vi "Red Pitaya Manager.vi"() -> ()   [LabVIEW 2024]
uses:
  Libraries/Red Pitaya/RP Core/RP Communicator/RP Communicator.lvclass
  <vilib>/regexp/Match Regular Expression.xnode
  Libraries/Red Pitaya/Red Pitaya Digitizer/Red Pitaya Digitizer.lvclass
  Libraries/Red Pitaya/RP Command.ctl
  Libraries/Red Pitaya/RP Status Offsets.ctl
  Libraries/Red Pitaya/RP Config Offsets.ctl
  Libraries/Red Pitaya/RP Channel Calibration.ctl
  Libraries/Red Pitaya/RP Calibration 4ch.ctl
  Libraries/Red Pitaya/RP Channel Filter.ctl
  Libraries/Red Pitaya/RP Filter 4ch.ctl
  Libraries/Red Pitaya/RP Calibration 2ch.ctl
  Libraries/Red Pitaya/RP Calibration.ctl
panel:
  in  "minimized shell":bool
  in  "Find Red Pitayas":bool
  out "Calibration":T1
  out "output cluster":T1
  in  "Tab Control":enum32{"Manage", "Settings", "Diagnostics"}(tab)
  out "String":string
  in  "Calibration string":bool
  in  "Applied \nvoltage":dbl=0.5
  in  "Auto gains":bool
  in  "Auto offsets":bool
  in  "Out amplitude":dbl[](array[numeric])=[0.5, 0.5]
  in  "Frequencies":dbl[](array[numeric])=[0.0, 0.0] format="%#_6pHz"
  in  "Out enable":bool[](array[boolean])
  in  "Out gains":dbl[](array[numeric])=[1.0, 1.0]
  in  "Out offsets":i16[](array[numeric])=[0, 0]
  in  "Reset calibration":bool
  out "Waveform Chart":dbl[][](graph)
  in  "Input ranges":bool[](array[boolean])=[FALSE, FALSE, FALSE, FALSE]
  in  "In offsets":i32[](array[numeric])
  in  "In gains":dbl[](array[numeric])
  out "Calibrating":bool
  in  "Write callibration":bool
  in  "Stop calibration":bool
  in  "Start calibration":bool
  out "Starup script":string
  in  "View  startup":bool
  in  "View  bitfiles":bool
  in  "Red Pitayas":i32(listbox)
  out "bit files":string
  in  "bitfile functionality":string[](array[string])=["variable-rate digitizer", "lockin-digitizer", "slow lockin-digitizer", "lockin-digitizer  for 122.88", "fast 4-ch digitizer", "critical current", "slow critical current", "variable rate 4-ch digitizer", "slow I-V v.7020"]
  in  "Bitfile logic tags 2":u16[](array[numeric])=[152, 159, 164, 169, 157, 154, 155, 158, 156]
  in  "Subnet":string="192.168.1"
  in  "Start address":i32=100
  in  "End address":i32=123
  in  "Bitfile logic tags":u16[](array[numeric])=[101, 102, 109, 113, 152, 154, 155, 156, 157, 158, 159, 164, 169]
  in  "Timeout":i32=100
  out "Bitfile IDs map":map{u16, string}(c390)={152="variable-rate digitizer", 154="critical current", 155="slow critical current", 157="fast 4-ch digitizer", 159="lockin-digitizer", 164="slow lockin-digitizer", 169="lockin-digitizer  for 122.88"}
  out "Addresses":string[](array[string])
  out "Device names":string[](array[string])
  out "Modules":i32[](array[numeric])
  out "DDS modula out":i64[](array[numeric])=[101, 102]
  out "Logic tags out":u16[](array[numeric])=[101, 102]
  out "command":string
  in  "error in":errorcluster
  out "error out":errorcluster
  in  "Exit Button":bool
  # "Input calibration"
  # "Output calibration"
  # "typedef enum {\n    STEM_125_10_v1_0            = 0,\n    STEM_125_14_v1_0            = 1,\n    STEM_125_14_v1_1            = 2,\n    STEM_122_16SDR_v1_0         = 3,\n    STEM_122_16SDR_v1_1         = 4,\n    STEM_125_14_LN_v1_1         = 5,\n    STEM_125_14_Z7020_v1_0      = 6,\n    STEM_125_14_Z7020_LN_v1_1   = 7,\n    STEM_125_14_Z7020_4IN_v1_0  = 8,\n    STEM_125_14_Z7020_4IN_v1_2  = 9,\n    STEM_125_14_Z7020_4IN_v1_3  = 10,\n    STEM_250_12_v1_0            = 11,\n    STEM_250_12_v1_1            = 12,\n    STEM_250_12_v1_2            = 13,\n    STEM_250_12_120             = 14,\n    STEM_250_12_v1_2a           = 15,\n    STEM_250_12_v1_2b           = 16,\n    STEM_125_14_LN_BO_v1_1      = 17,\n    STEM_125_14_LN_CE1_v1_1     = 18,\n    STEM_125_14_LN_CE2_v1_1     = 19\n}  rp_HPeModels_t;"
  # "typedef enum {\n    Z7010 = 0,\n    Z7020 = 1\n}  rp_HPeZynqModels_t;"
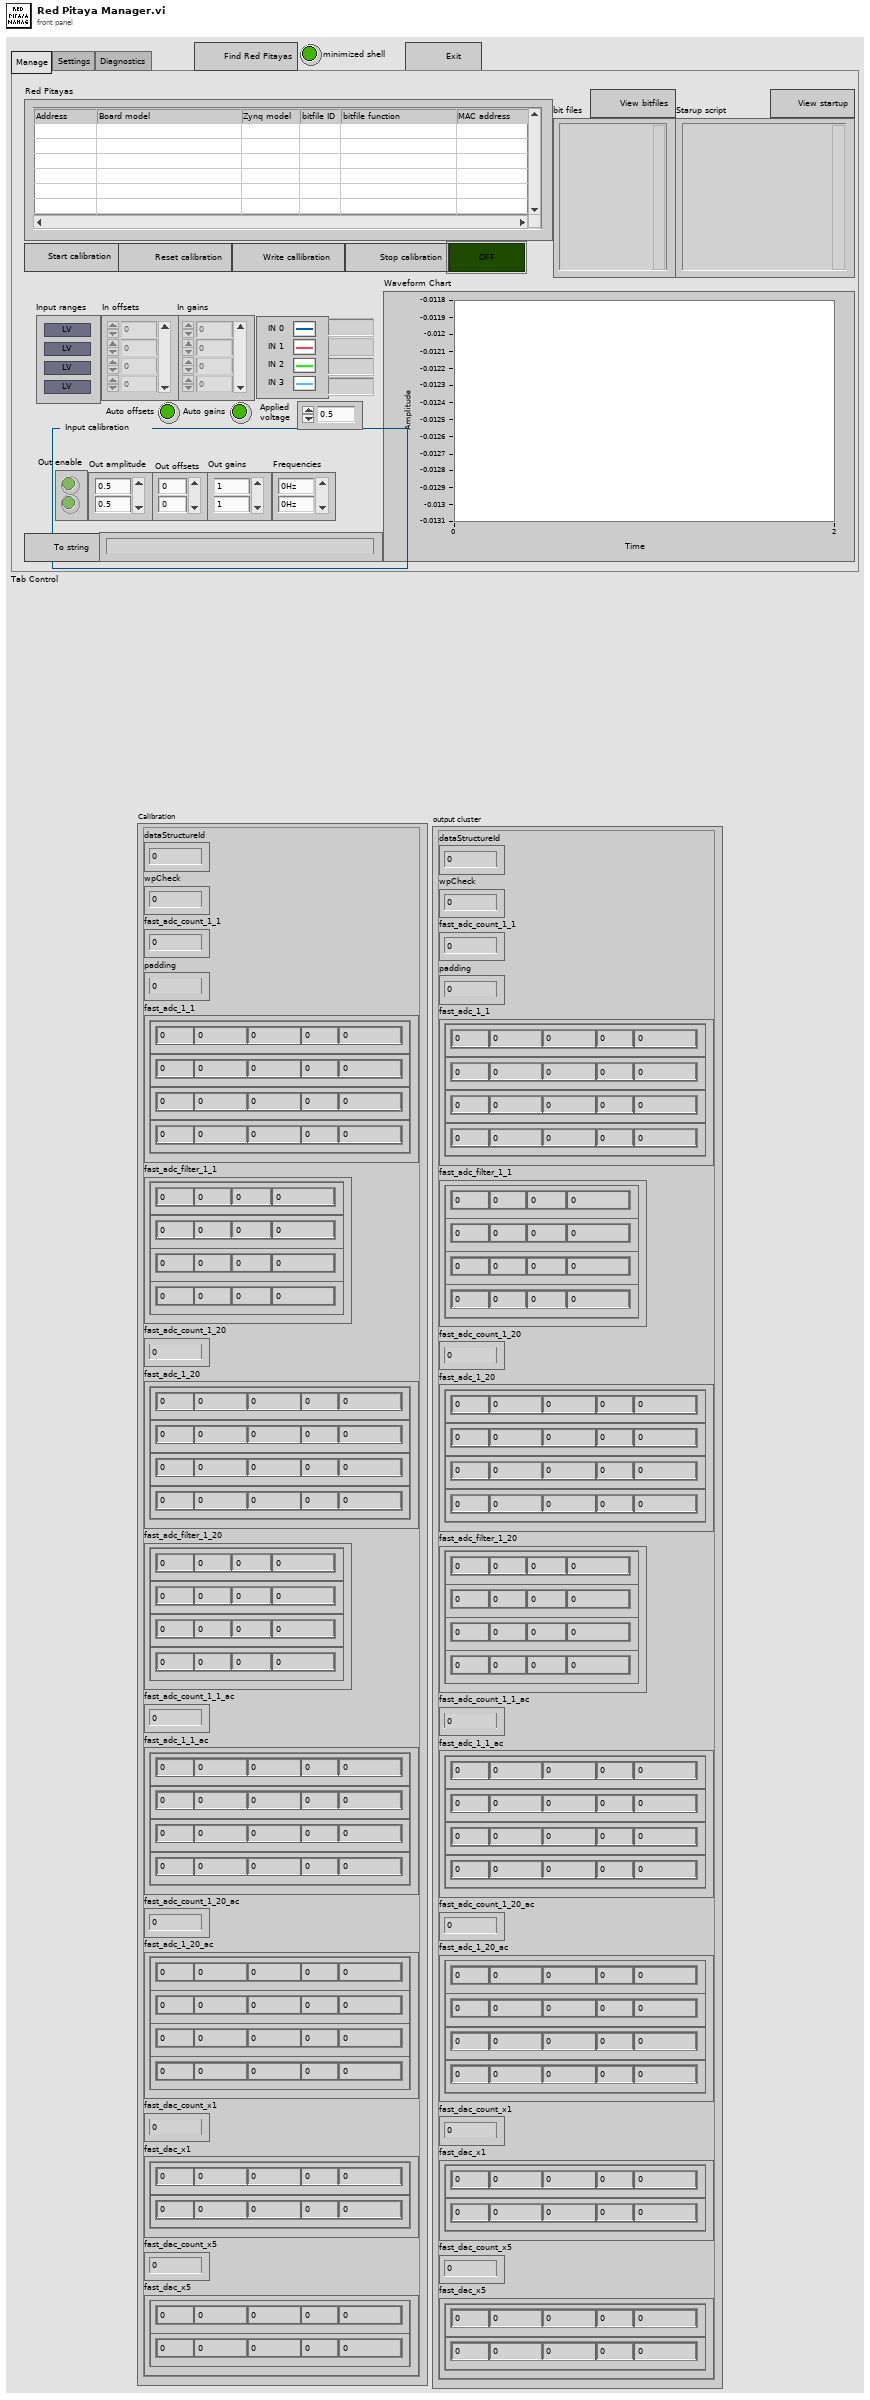
[diagram p1: front panel]
types:
  T1 = typedef "RP Calibration.ctl" = cluster{"dataStructureId":u8, "wpCheck":u8, "fast_adc_count_1_1":u16, "padding":u32, "fast_adc_1_1":T2, "fast_adc_filter_1_1":T4, "fast_adc_count_1_20":u64, "fast_adc_1_20":T2, "fast_adc_filter_1_20":T4, "fast_adc_count_1_1_ac":u64, "fast_adc_1_1_ac":T2, "fast_adc_count_1_20_ac":u64, "fast_adc_1_20_ac":T2, "fast_dac_count_x1":u64, "fast_dac_x1":T6, "fast_dac_count_x5":u64, "fast_dac_x5":T6}
  T2 = typedef "RP Calibration 4ch.ctl" = cluster{"ch_0":T3, "ch_1":T3, "ch_2":T3, "ch_3":T3}
  T3 = typedef "RP Channel Calibration.ctl" = cluster{"baseScale":sgl, "calibValue":u32, "offset":i32, "padding 2":i32, "gainCalc":dbl}
  T4 = typedef "RP Filter 4ch.ctl" = cluster{"ch_0":T5, "ch_1":T5, "ch_2":T5, "ch_3":T5}
  T5 = typedef "RP Channel Filter.ctl" = cluster{"aa":u32, "bb":u32, "pp":u32, "kk":u32}
  T6 = typedef "RP Calibration 2ch.ctl" = cluster{"ch_0":T3, "ch_1":T3}
  T7 = typedef "RP Command.ctl" = enum16{"Reset", "Read IDN", "Stop server", "Get status", "Get temperature", "Connect client", "Arm", "Software trigger", "Get whole buffer", "Get chunk", "System call", "Get config", "Set config", "Recieve data", "Recieve Calibartion", "Transmit data"}
  T8 = typedef "RP Config Offsets.ctl" = u16
  T9 = typedef "RP Status Offsets.ctl" = u16
  T10 = cluster{"fast_dac_x1[0]":T3, "fast_dac_x1[1]":T3}
  T11 = cluster{"fast_adc_1_1[0]":T3, "fast_adc_1_1[1]":T3, "fast_adc_1_1[2]":T3, "fast_adc_1_1[3]":T3}
  T12 = cluster{"fast_adc_1_20[0]":T3, "fast_adc_1_20[1]":T3, "fast_adc_1_20[2]":T3, "fast_adc_1_20[3]":T3}
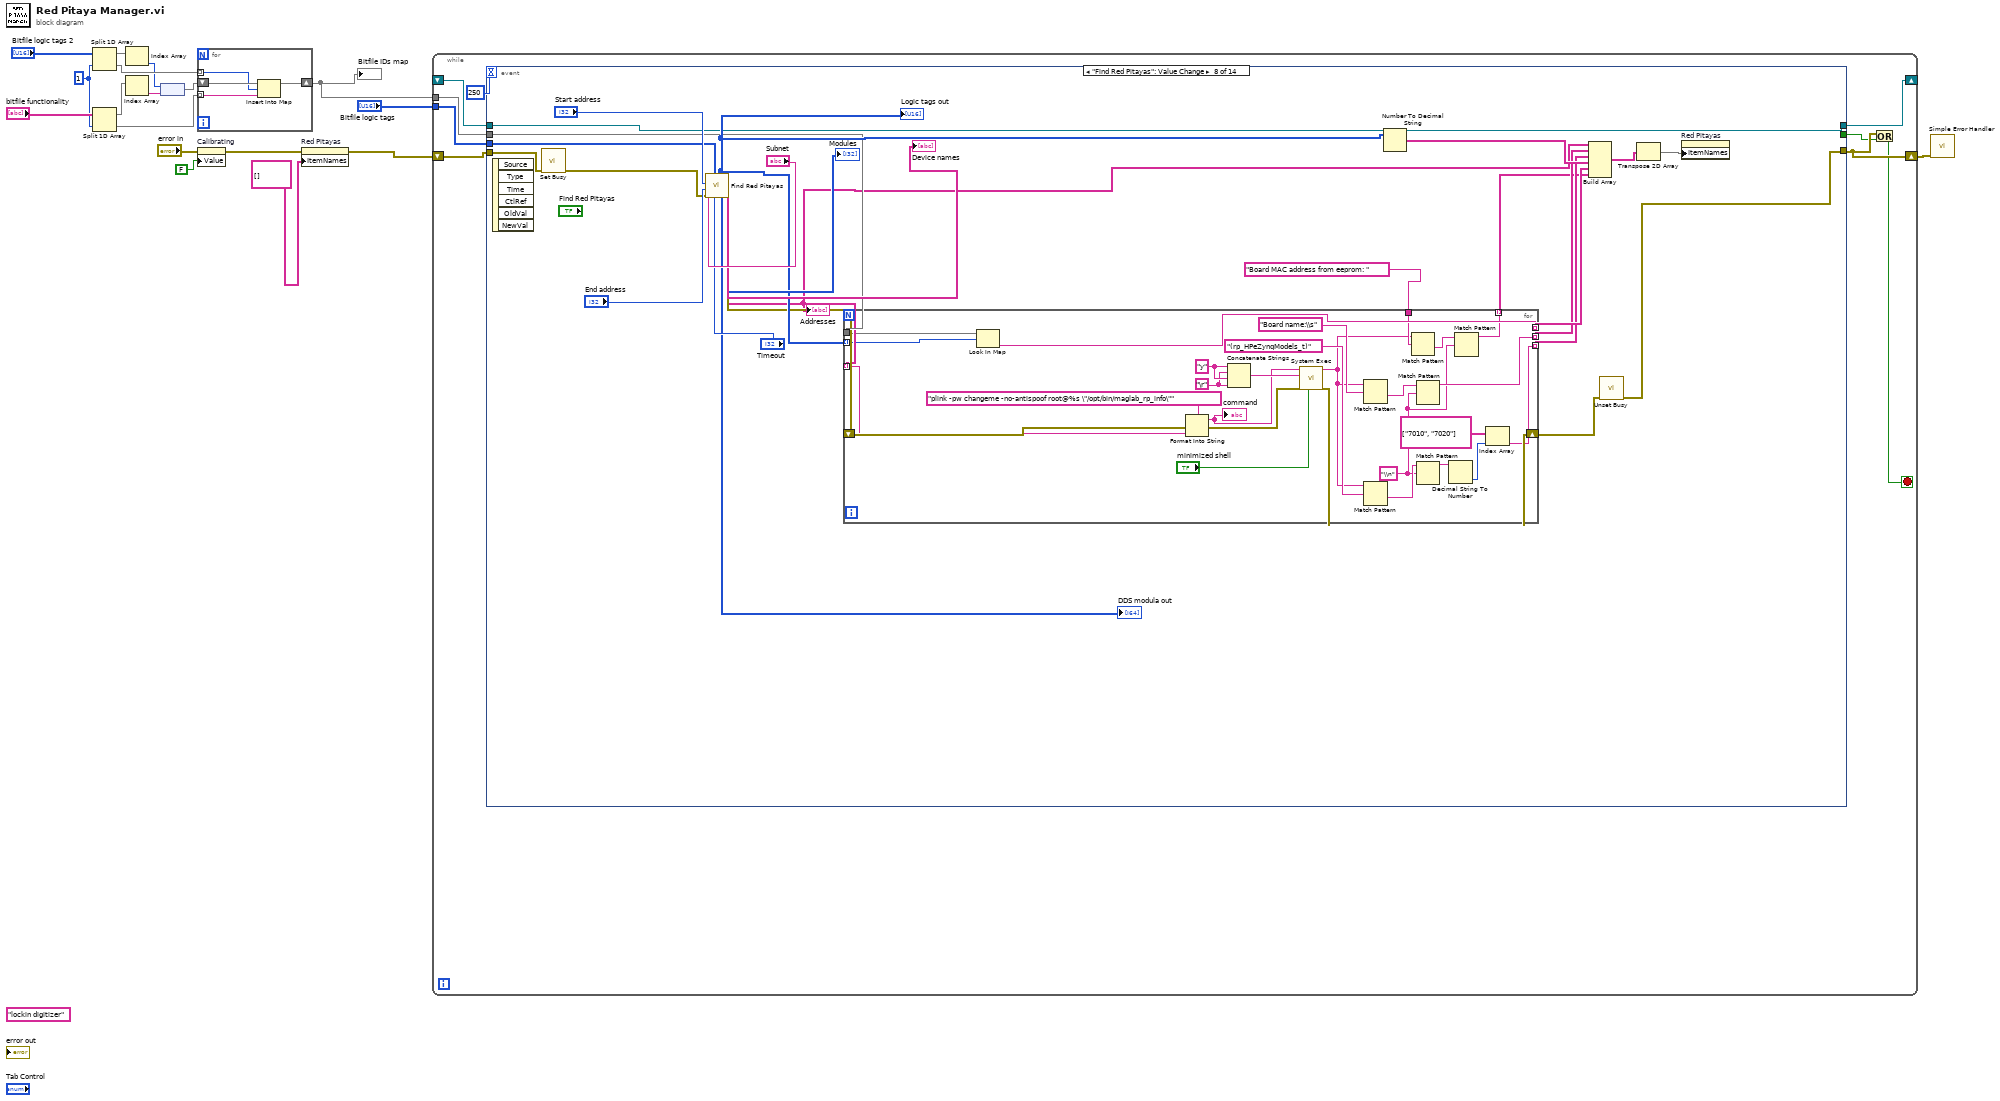
[diagram p0: block diagram]
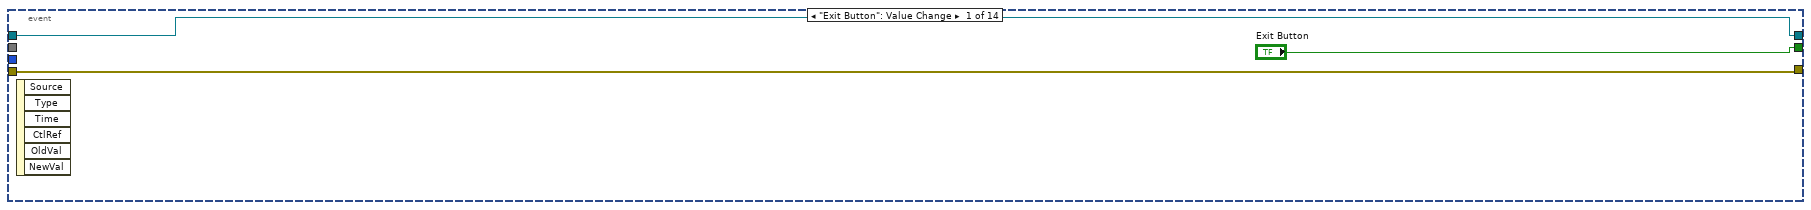
[diagram p2: hidden frame]
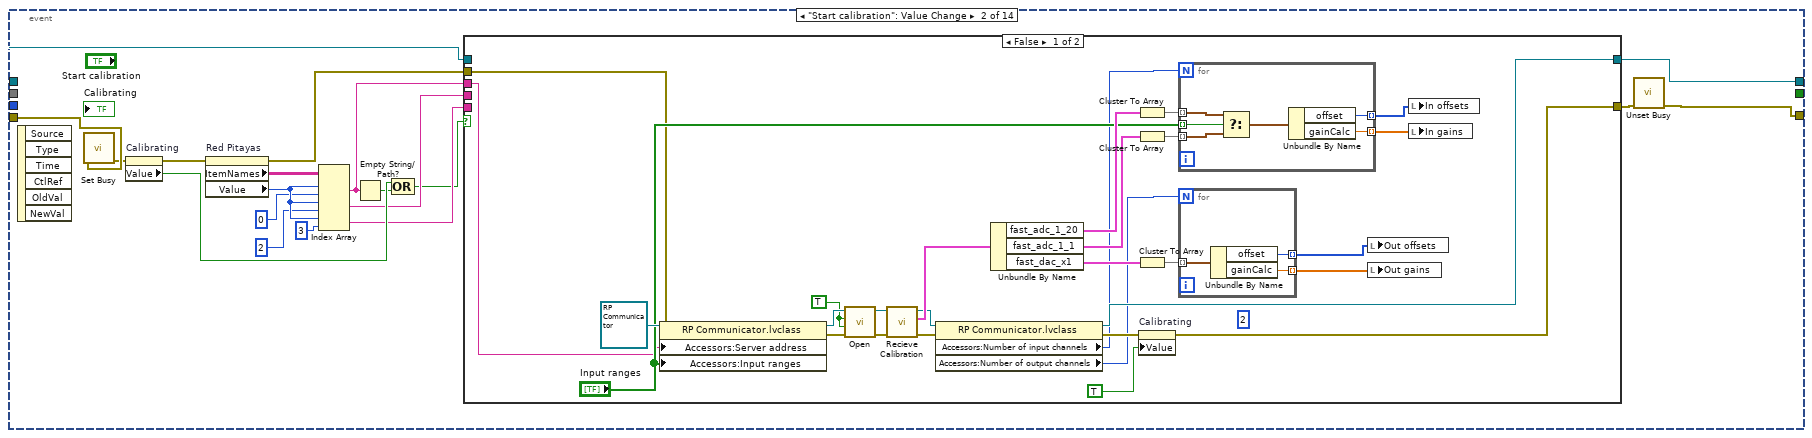
[diagram p3: hidden frame]
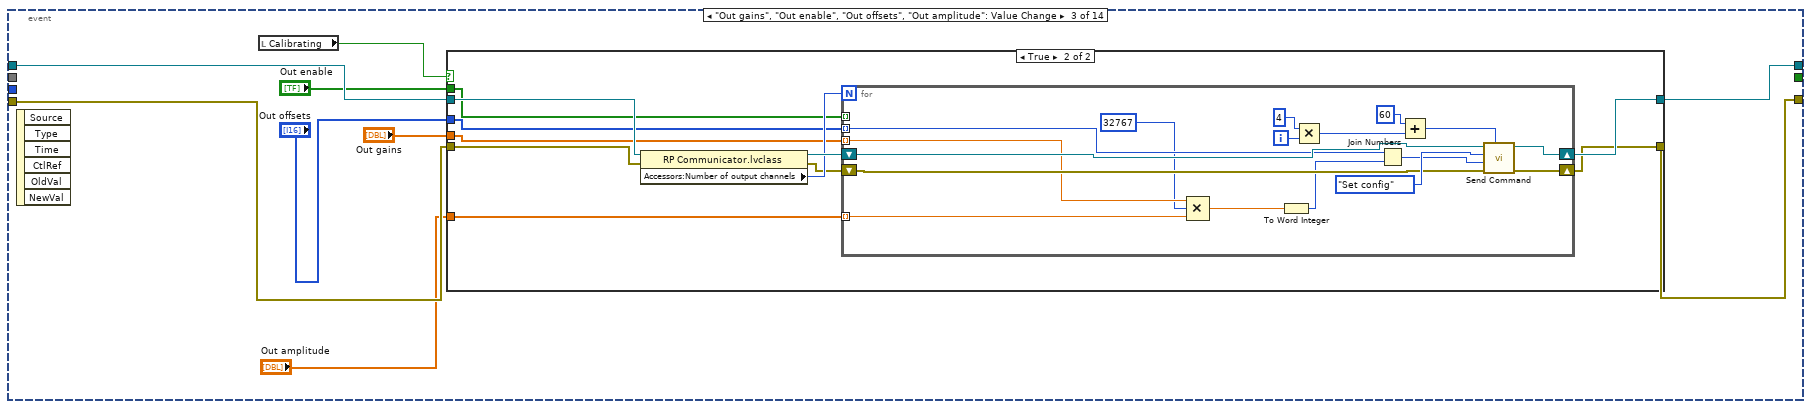
[diagram p5: hidden frame]
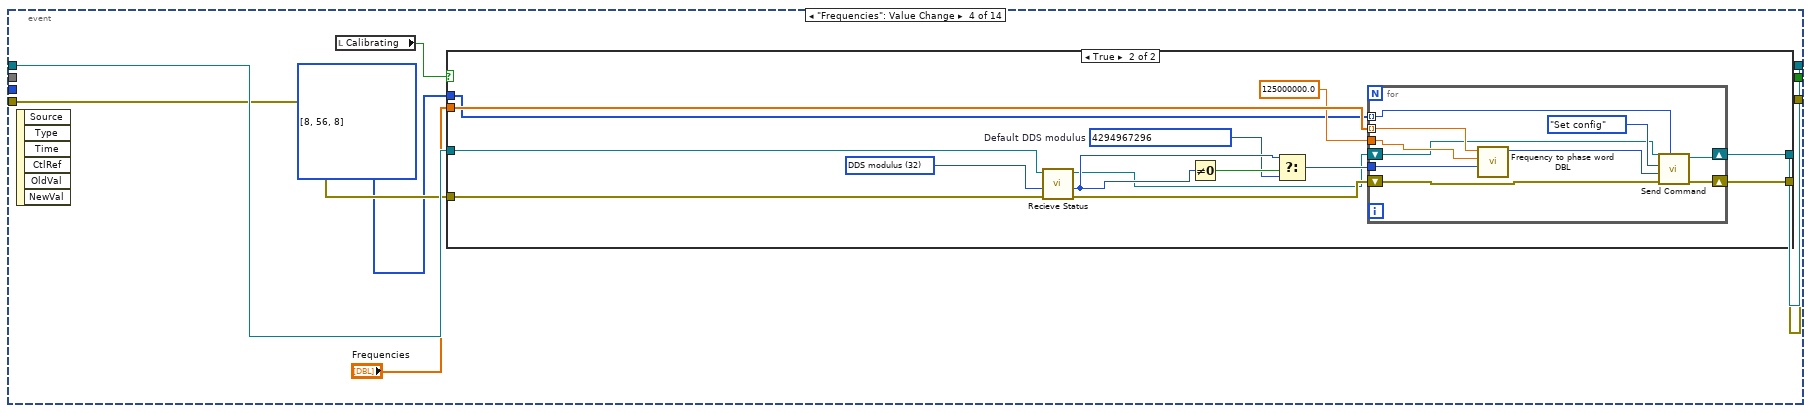
[diagram p7: hidden frame]
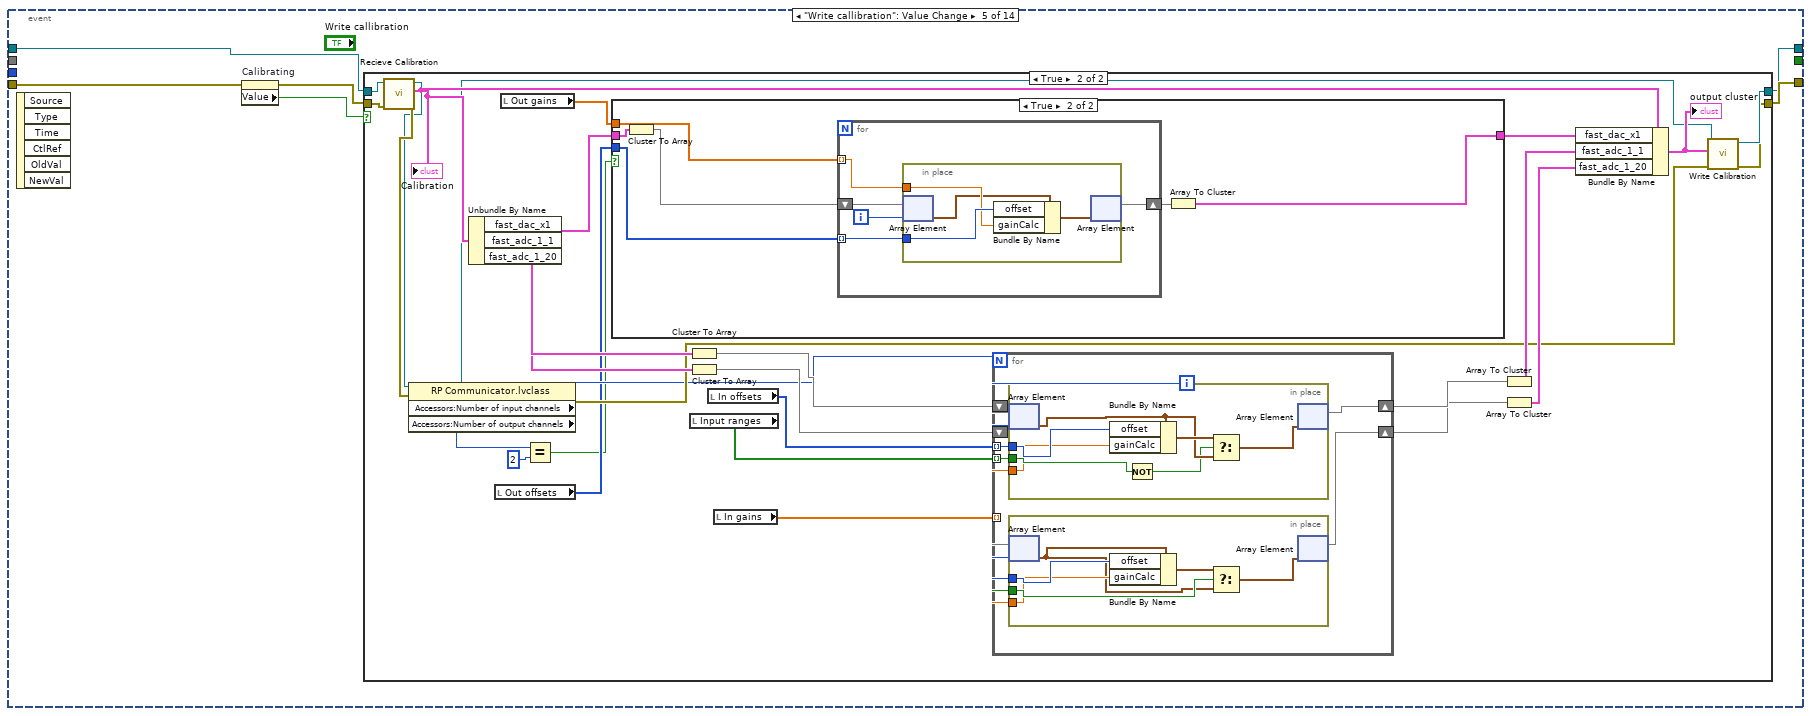
[diagram p9: hidden frame]
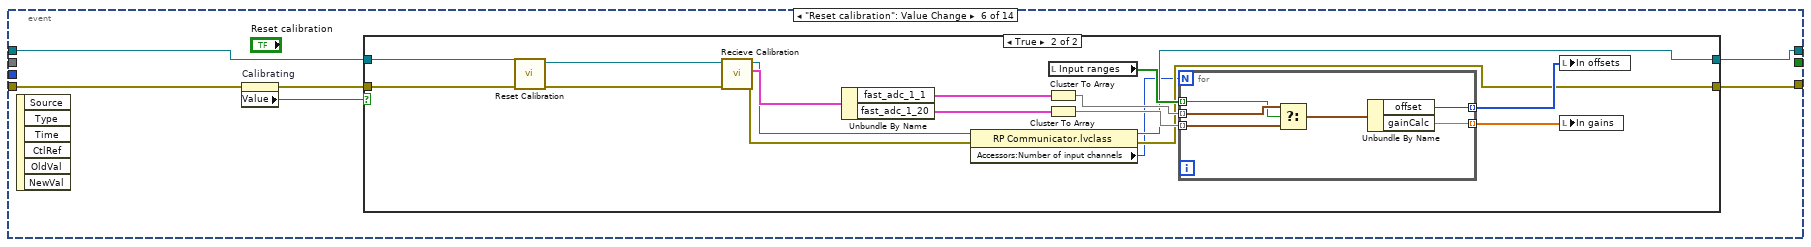
[diagram p12: hidden frame]
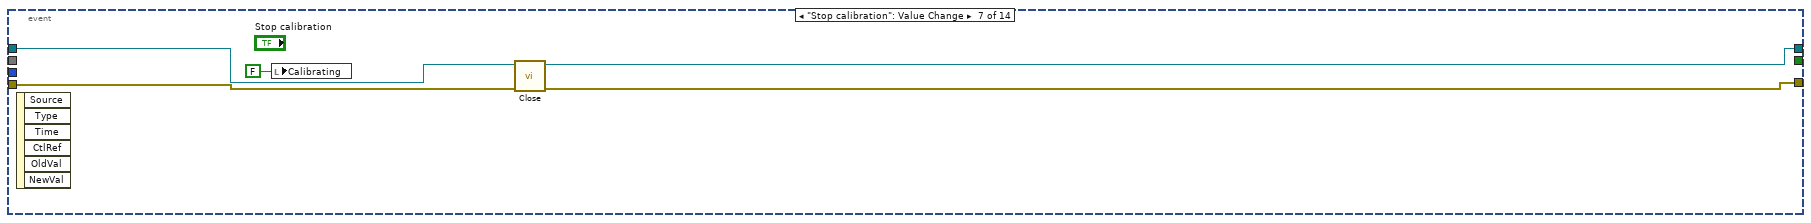
[diagram p14: hidden frame]
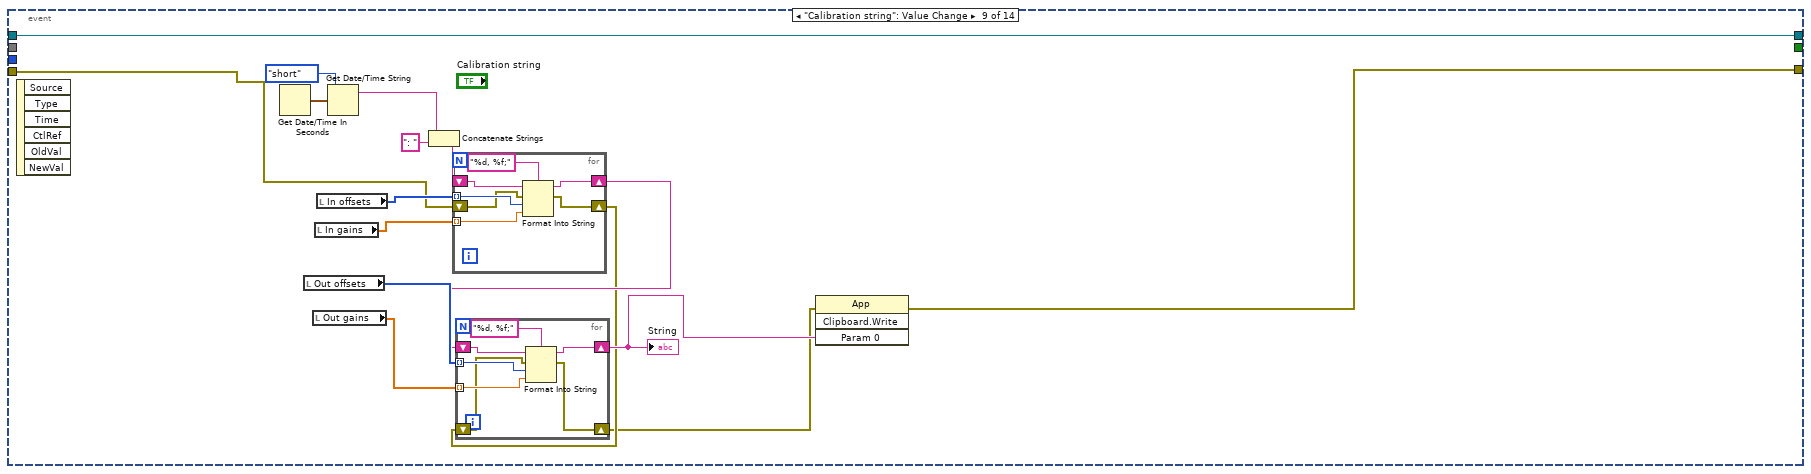
[diagram p15: hidden frame]
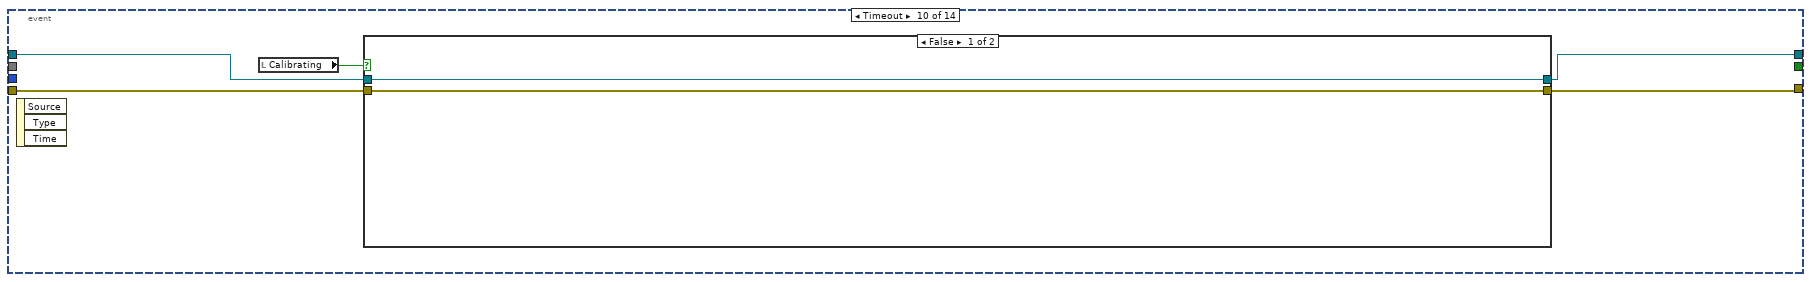
[diagram p16: hidden frame]
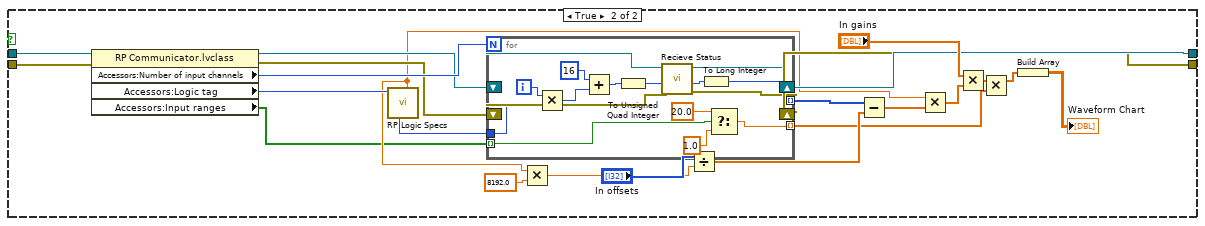
[diagram p17: hidden frame]
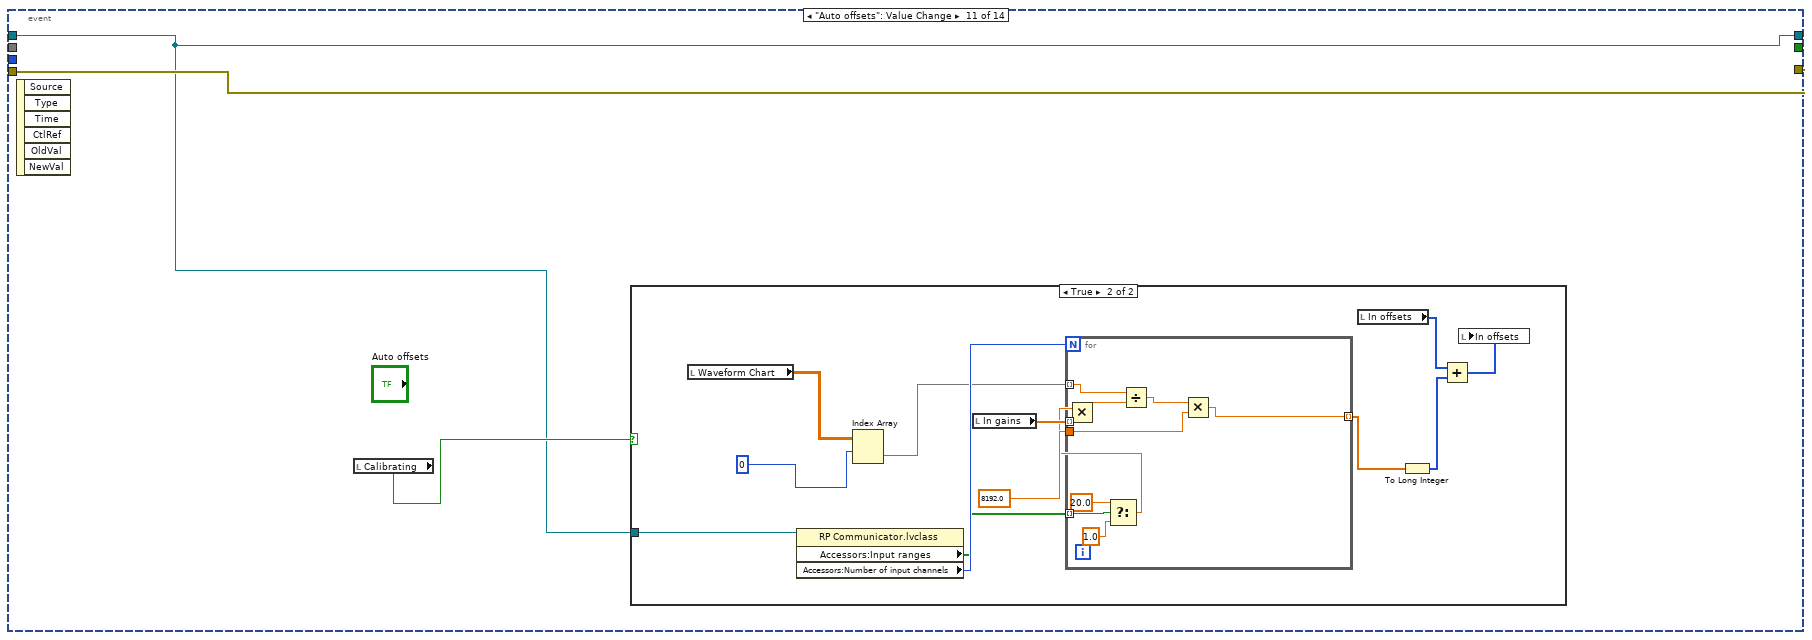
[diagram p18: hidden frame]
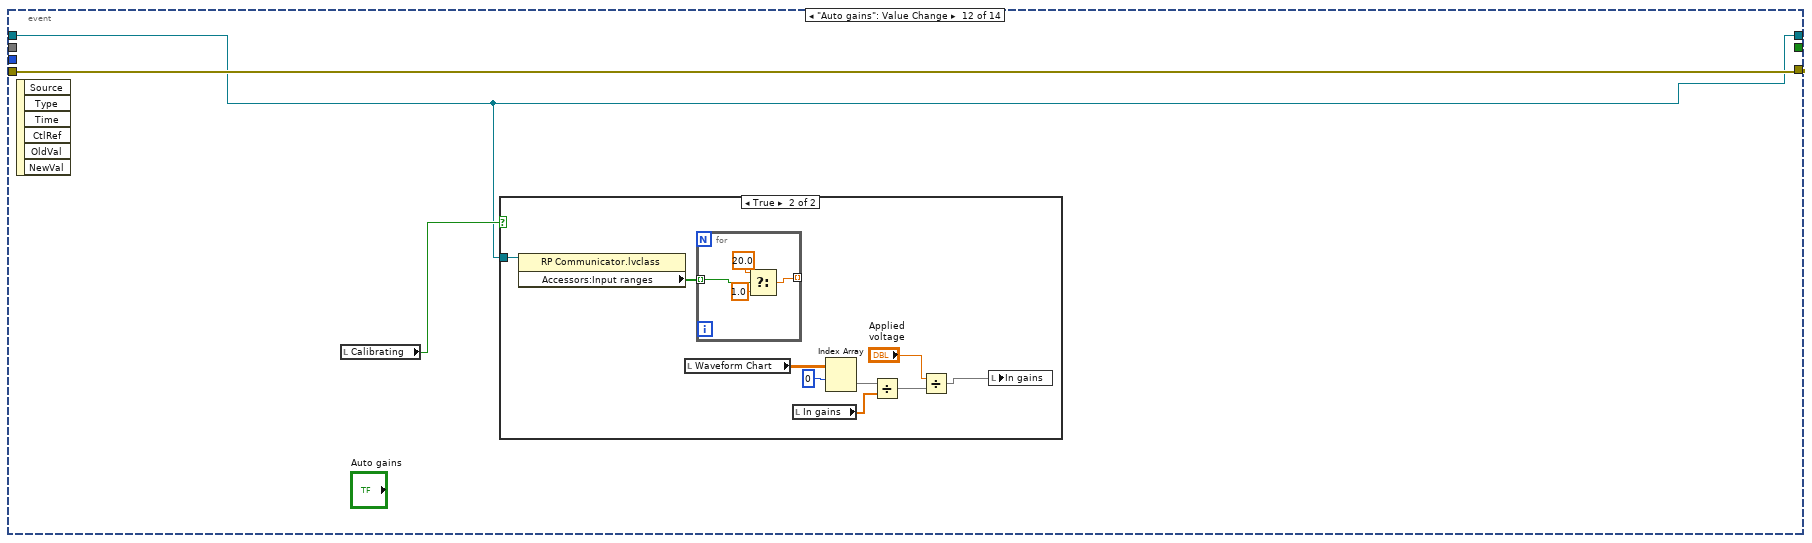
[diagram p20: hidden frame]
diagram:
  w15 = 1 ("index")
  (unwired) "lockin digitizer" ("value")
  n1 = Split 1D Array(array="Bitfile logic tags 2", index=w15) -> (first subarray=w14:u16[], second subarray=w12:u16[])
  n2 = Split 1D Array(array="bitfile functionality", index=w15) -> (first subarray=w13:string[], second subarray=w11:string[])
  n3 = Index Array(array=w14) -> (element=w9:u16)  [unwired: 1 in]
  n4 = Index Array(array=w13) -> (element=w8:string)  [unwired: 1 in]
  n5 = node(w9, w8) -> (w10:map{u16, string})
  n6 = for {
    tunnel: w12 -> [w21] mode=indexing
    tunnel: w11 -> [w20] mode=indexing
    shift-right: [w19] -> w7
    shift-left: w10 -> [w22]
    n7 = Insert Into Map(map in=w22, key=w21, value=w20) -> (map out=w19:map{u16, string})  [unwired: 2 out]
  }
  "Bitfile IDs map" <- w7
  n8 = property on="Calibrating" class="Bool (strict)"(error in="error in", "Value"=FALSE ("Calibrating")) -> (error out=w2:errorcluster)  [unwired: 1 in, 1 out]
  n9 = property on="Red Pitayas" class="MCListbox (strict)"(error in=w2, "ItemNames"=string[][] [] ("Item Names")) -> (error out=w1:errorcluster)  [unwired: 1 in, 1 out]
  n10 = while {
    tunnel: "Bitfile logic tags" -> [w31]
    tunnel: w7 -> [w30]
    shift-right: [w27] -> w6
    shift-left: w1 -> [w29]
    shift-right: [w24] -> _
    shift-left: _ -> [w23]
    stop <- w25 stop-if-true
    n11 = event shown="[7] \"Find Red Pitayas\": Value Change" {
      selector: _ -> [_ _ _ _ _ _ _ _ _ _ _ _ _ _]
      dyn-events: _ -> [_ _ _ _ _ _ _ _ _ _ _ _ _ _]
      timeout: 250 -> [_ _ _ _ _ _ _ _ _ _ _ _ _ _]
      tunnel: ["Exit Button" _ _ _ _ _ _ _ _ _ _ _ _ _] -> w26
      tunnel: w31 -> [_ _ _ _ _ _ _ w289 _ _ _ _ _ _]
      tunnel: w30 -> [_ _ _ _ _ _ _ w287 _ _ _ _ _ _]
      tunnel: w29 -> [w33 w51 w100 w134 w170 w244 w270 w281 w335 w360 w404 w430 w454 w596]
      tunnel: [w33 w35 w99 w135 w166 w240 w271 w279 w332 w359 w404 w430 w444 w590] -> w27
      tunnel: [w32 w52 w97 w136 w165 w239 w273 w277 w336 w357 w403 w428 w448 w592] -> w24
      tunnel: w23 -> [w32 w49 w98 w137 w168 w241 w272 w277 w336 w358 w403 w428 w448 w592]
      event "Exit Button": Value Change {
        n12 = event-data() -> ()  [unwired: 1 in, 6 out]
      }
      event "Start calibration": Value Change {
        n13 = event-data() -> ()  [unwired: 1 in, 6 out]
        n14 = call <vilib>:"Set Busy.vi"("error in (no error)"=w51) -> ("error out"=w36:errorcluster)  [unwired: 9 in, 1 out]
        n15 = property on="Calibrating" class="Bool (strict)"(error in=w36) -> (error out=w41:errorcluster, "Value"=w50:bool)  [unwired: 1 in, 1 out]
        n16 = property on="Red Pitayas" class="MCListbox (strict)"(error in=w41) -> (error out=w40:errorcluster, "ItemNames"=w47:string[][], "Value"=w48:i32)  [unwired: 1 in, 1 out]
        n17 = Index Array(array=w47, index (row) #1=w48, index (col) #1=0 ("disabled index (col)"), index (row) #2=w48, index (col) #2=2 ("disabled index (col)"), index (row) #3=w48, index (col) #3=3 ("disabled index (col)")) -> (element #1=w38:string, element #2=w43:string, element #3=w42:string)
        n18 = Empty String/Path?(string/path=w38) -> (empty?=w37:bool)
        n19 = Compound Arithmetic op=OR(w50, w37) -> (w39:bool)
        n20 = case shown="False" w39 {
          tunnel: [w69 w92] -> w53
          tunnel: [w56 w91] -> w52
          tunnel: w40 -> [w66 w92]
          tunnel: w49 -> [_ w91]
          tunnel: w38 -> [w64 _]
          tunnel: w43 -> [_ _]
          tunnel: w42 -> [_ _]
          frame False {
            w59 = TRUE ("Send \"Connect client\"")
            (unwired) 2 ("Number of input channels")
            n21 = property class="RP Communicator.lvclass"(reference=refnum<class "RP Communicator.lvclass"> refnum ("RP Communicator.lvclass"), error in=w66, "Accessors:Server address"=w64, "Accessors:Input ranges"="Input ranges") -> (reference out=w67:refnum<class "RP Communicator.lvclass">, error out=w65:errorcluster)
            n22 = call-dynamic "Open.vi"("error in (no error)"=w65, "Read config"=w59, "Send \"Connect client\""=w59, "RP Communicator in"=w67) -> ("error out"=w80:errorcluster, "RP Communicator out"=w79:refnum<class "RP Communicator.lvclass">)  [unwired: 6 in]
            n23 = call-dynamic "Recieve Calibration.vi"("error in (no error)"=w80, "RP Communicator in"=w79) -> ("error out"=w70:errorcluster, "Calibration"=w78:T1, "RP Communicator out"=w57:refnum<class "RP Communicator.lvclass">)  [unwired: 7 in]
            n24 = property class="RP Communicator.lvclass"(reference=w57, error in=w70) -> (reference out=w56:refnum<class "RP Communicator.lvclass">, error out=w58:errorcluster, "Accessors:Number of input channels"=w55:i32, "Accessors:Number of output channels"=w54:i32)
            n25 = Unbundle By Name(w78) -> ("fast_adc_1_20"=w77:T2, "fast_adc_1_1"=w76:T2, "fast_dac_x1"=w63:T6)
            n26 = Cluster To Array(cluster=w77) -> (array=w75:T3[])
            n27 = Cluster To Array(cluster=w76) -> (array=w74:T3[])
            n28 = Cluster To Array(cluster=w63) -> (array=w62:T3[])
            n29 = property on="Calibrating" class="Bool (strict)"(error in=w58, "Value"=TRUE ("Calibrating")) -> (error out=w69:errorcluster)  [unwired: 1 in, 1 out]
            n30 = for {
              N: w55 -> [_]
              tunnel: w75 -> [w90] mode=indexing
              tunnel: w74 -> [w89] mode=indexing
              tunnel: "Input ranges" -> [w88] mode=indexing
              tunnel: [w86] -> w71 mode=indexing
              tunnel: [w85] -> w72 mode=indexing
              n31 = Select(t=w90, s=w88, f=w89) -> (s? t:f=w87:T3)
              n32 = Unbundle By Name(w87) -> ("offset"=w85:i32, "gainCalc"=w86:dbl)
            }
            n33 = for {
              N: w54 -> [_]
              tunnel: w62 -> [w84] mode=indexing
              tunnel: [w83] -> w60 mode=indexing
              tunnel: [w82] -> w61 mode=indexing
              n34 = Unbundle By Name(w84) -> ("offset"=w83:i32, "gainCalc"=w82:dbl)
            }
            n35 = local write "Out offsets"(w60) -> ()
            n36 = local write "Out gains"(w61) -> ()
            n37 = local write "In offsets"(w72) -> ()
            n38 = local write "In gains"(w71) -> ()
          }
          frame True {
          }
        }
        n39 = call <vilib>:"Unset Busy.vi"("error in (no error)"=w53) -> ("error out"=w35:errorcluster)  [unwired: 10 in]
      }
      event "Out gains", "Out enable", "Out offsets", "Out amplitude": Value Change {
        n40 = event-data() -> ()  [unwired: 1 in, 6 out]
        n41 = local read "Calibrating"() -> (w101:bool)
        n42 = case shown="True" w101 {
          tunnel: w100 -> [w103 w110]
          tunnel: [w103 w108] -> w99
          tunnel: w98 -> [w102 w114]
          tunnel: [w102 w113] -> w97
          tunnel: "Out offsets" -> [_ w107]
          tunnel: "Out enable" -> [_ w106]
          tunnel: "Out gains" -> [_ w105]
          tunnel: "Out amplitude" -> [_ w104]
          frame False {
          }
          frame True {
            n43 = property class="RP Communicator.lvclass"(reference=w114, error in=w110) -> (reference out=w112:refnum<class "RP Communicator.lvclass">, error out=w109:errorcluster, "Accessors:Number of output channels"=w111:i32)
            n44 = for {
              N: w111 -> [_]
              tunnel: w106 -> [_] mode=indexing
              tunnel: w107 -> [w118] mode=indexing
              tunnel: w105 -> [w121] mode=indexing
              shift-right: [w130] -> w113
              shift-left: w112 -> [w131]
              shift-right: [w122] -> w108
              shift-left: w109 -> [w123]
              tunnel: w104 -> [w115] mode=indexing
              i -> [w126]
              n45 = Compound Arithmetic op=MULTIPLY(w121, i16 32767, w115) -> (w120:dbl)
              n46 = To Word Integer(number=w120) -> (16bit integer=w119:i16)
              n47 = Multiply(x=4, y=w126) -> (x*y=w125:i32)
              n48 = Join Numbers(hi=w118, lo=w119) -> ((hi.lo)=w117:u32)
              n49 = Add(x=60, y=w125) -> (x+y=w124:i32)
              n50 = call-dynamic "Send Command.vi"("Config offset"=w124, "error in (no error)"=w123, "Command payload"=w117, "Command number"=RP_Command."Set config", "RP Communicator in"=w131) -> ("error out"=w122:errorcluster, "RP Communicator out"=w130:refnum<class "RP Communicator.lvclass">)  [unwired: 4 in, 1 out]
            }
          }
        }
      }
      event "Frequencies": Value Change {
        w132 = T8[] [8, 56, 8] items=["Config flags"=0, "Record length"=4, "Frequency 0"=8, "Decimation"=12, "LED"=16, "DDS delay"=28, "Fequency 1"=56]
        n51 = event-data() -> ()  [unwired: 1 in, 6 out]
        n52 = local read "Calibrating"() -> (w138:bool)
        n53 = case shown="True" w138 {
          tunnel: w137 -> [w140 w152]
          tunnel: [w140 w143] -> w136
          tunnel: [w139 w142] -> w135
          tunnel: w134 -> [w139 w151]
          tunnel: "Frequencies" -> [_ w154]
          tunnel: w132 -> [_ w141]
          frame False {
          }
          frame True {
            w147 = i64 4294967296  # Default DDS modulus
            w150 = T9 32 items=["Writer address"=0, "Record start position"=4, "Trig state and ID"=8, "Phase"=12, "X1"=16, "Y1"=20, "RxFIFO counter or  X2"=24, "TxFIFO counter or Y2"=28, "DDS modulus"=32] ("Status offsets")
            n54 = call-dynamic "Recieve Status.vi"("error in (no error)"=w151, "Status offset"=w150, "RP Communicator in"=w152) -> ("error out"=w145:errorcluster, "Status response"=w148:u32, "RP Communicator out"=w144:refnum<class "RP Communicator.lvclass">)  [unwired: 6 in]
            n55 = Not Equal To 0?(x=w148) -> (x != 0?=w149:bool)
            n56 = Select(t=w148, s=w149, f=w147) -> (s? t:f=w146:i64)
            n57 = for {
              tunnel: w154 -> [w164] mode=indexing
              tunnel: 125000000.0 ("DDS clock") -> [w163]
              tunnel: w146 -> [w162]
              shift-right: [w157] -> w142
              shift-left: w145 -> [w161]
              shift-right: [w158] -> w143
              shift-left: w144 -> [w159]
              tunnel: w141 -> [w156] mode=indexing
              n58 = call "Frequency to phase word DBL.vi"("DDS modulus"=w162, "DDS clock"=w163, "Frequency"=w164) -> ("Phase word"=w155:u64)  [unwired: 7 in, 1 out]
              n59 = call-dynamic "Send Command.vi"("Config offset"=w156, "error in (no error)"=w161, "Command payload"=w155, "Command number"=RP_Command."Set config", "RP Communicator in"=w159) -> ("error out"=w157:errorcluster, "RP Communicator out"=w158:refnum<class "RP Communicator.lvclass">)  [unwired: 4 in, 1 out]
            }
          }
        }
      }
      event "Write callibration": Value Change {
        n60 = event-data() -> ()  [unwired: 1 in, 6 out]
        n61 = property on="Calibrating" class="Bool (strict)"(error in=w170) -> (error out=w167:errorcluster, "Value"=w169:bool)  [unwired: 1 in, 1 out]
        n62 = case shown="True" w169 {
          tunnel: w168 -> [w172 w201]
          tunnel: w167 -> [w171 w200]
          tunnel: [w171 w185] -> w166
          tunnel: [w172 w187] -> w165
          frame False {
          }
          frame True {
            n63 = call-dynamic "Recieve Calibration.vi"("error in (no error)"=w200, "RP Communicator in"=w201) -> ("error out"=w186:errorcluster, "Calibration"=w191:T1, "RP Communicator out"=w182:refnum<class "RP Communicator.lvclass">)  [unwired: 7 in]
            "Calibration" <- w191
            n64 = property class="RP Communicator.lvclass"(reference=w182, error in=w186) -> (reference out=w181:refnum<class "RP Communicator.lvclass">, error out=w183:errorcluster, "Accessors:Number of input channels"=w180:i32, "Accessors:Number of output channels"=w177:i32)
            n65 = Unbundle By Name(w191) -> ("fast_dac_x1"=w173:T6, "fast_adc_1_1"=w196:T2, "fast_adc_1_20"=w195:T2)
            n66 = local read "Out offsets"() -> (w179:i16[])
            n67 = local read "Out gains"() -> (w178:dbl[])
            n68 = Equal?(x=w177, y=2) -> (x = y?=w175:bool)
            n69 = case shown="True" w175 {
              tunnel: w173 -> [w202 w208]
              tunnel: w179 -> [_ w206]
              tunnel: w178 -> [_ w205]
              tunnel: [w202 w203] -> w174
              frame False {
              }
              frame True {
                n70 = Cluster To Array(cluster=w208) -> (array=w207:T3[])
                n71 = for {
                  tunnel: w206 -> [w213] mode=indexing
                  tunnel: w205 -> [w212] mode=indexing
                  shift-right: [w209] -> w204
                  shift-left: w207 -> [w211]
                  i -> [w210]
                  n72 = in-place {
                    in-place-border: w213 -> [w217]
                    in-place-border: w212 -> [w216]
                    n73 = in-place-array #1(w211, w210) -> (w215:T3)
                    n74 = Bundle By Name(cluster=w215, "offset"=w217, "gainCalc"=w216) -> (w214:T3)
                    n75 = in-place-array #1(w214) -> (w209:T3[])  [unwired: 1 out]
                  }
                }
                n76 = Array To Cluster(array=w204) -> (cluster=w203:T10)
              }
            }
            n77 = Cluster To Array(cluster=w196) -> (array=w194:T3[])
            n78 = Cluster To Array(cluster=w195) -> (array=w193:T3[])
            n79 = local read "Input ranges"() -> (w199:bool[])
            n80 = local read "In offsets"() -> (w198:i32[])
            n81 = local read "In gains"() -> (w197:dbl[])
            n82 = for {
              N: w180 -> [_]
              tunnel: w199 -> [w224] mode=indexing
              tunnel: w198 -> [w223] mode=indexing
              tunnel: w197 -> [w222] mode=indexing
              shift-right: [w219] -> w192
              shift-left: w194 -> [w225]
              shift-right: [w218] -> w189
              shift-left: w193 -> [w221]
              i -> [w220]
              n83 = in-place {
                in-place-border: w224 -> [w231]
                in-place-border: w223 -> [w230]
                in-place-border: w222 -> [w229]
                n84 = in-place-array #2(w225, w220) -> (w227:T3)
                n85 = Bundle By Name(cluster=w227, "offset"=w230, "gainCalc"=w229) -> (w232:T3)
                n86 = Not(x=w231) -> (.not. x?=w226:bool)
                n87 = Select(t=w232, s=w226, f=w227) -> (s? t:f=w228:T3)
                n88 = in-place-array #2(w228) -> (w219:T3[])  [unwired: 1 out]
              }
              n89 = in-place {
                in-place-border: w224 -> [w238]
                in-place-border: w223 -> [w237]
                in-place-border: w222 -> [w236]
                n90 = in-place-array #3(w221, w220) -> (w234:T3)
                n91 = Bundle By Name(cluster=w234, "offset"=w237, "gainCalc"=w236) -> (w233:T3)
                n92 = Select(t=w233, s=w238, f=w234) -> (s? t:f=w235:T3)
                n93 = in-place-array #3(w235) -> (w218:T3[])  [unwired: 1 out]
              }
            }
            n94 = Array To Cluster(array=w192) -> (cluster=w190:T11)
            n95 = Array To Cluster(array=w189) -> (cluster=w188:T12)
            n96 = Bundle By Name(cluster=w191, "fast_dac_x1"=w174, "fast_adc_1_1"=w190, "fast_adc_1_20"=w188) -> (w184:T1)
            "output cluster" <- w184
            n97 = call-dynamic "Write Calibration.vi"("error in (no error)"=w183, "Calibration"=w184, "RP Communicator in"=w181) -> ("error out"=w185:errorcluster, "RP Communicator out"=w187:refnum<class "RP Communicator.lvclass">)  [unwired: 7 in]
          }
        }
      }
      event "Reset calibration": Value Change {
        n98 = event-data() -> ()  [unwired: 1 in, 6 out]
        n99 = property on="Calibrating" class="Bool (strict)"(error in=w244) -> (error out=w242:errorcluster, "Value"=w243:bool)  [unwired: 1 in, 1 out]
        n100 = case shown="True" w243 {
          tunnel: w242 -> [w246 w263]
          tunnel: w241 -> [w245 w262]
          tunnel: [w246 w250] -> w240
          tunnel: [w245 w248] -> w239
          frame False {
          }
          frame True {
            n101 = call-dynamic "Reset Calibration.vi"("error in (no error)"=w263, "RP Communicator in"=w262) -> ("error out"=w256:errorcluster, "RP Communicator out"=w255:refnum<class "RP Communicator.lvclass">)  [unwired: 8 in]
            n102 = call-dynamic "Recieve Calibration.vi"("error in (no error)"=w256, "RP Communicator in"=w255) -> ("error out"=w252:errorcluster, "Calibration"=w261:T1, "RP Communicator out"=w249:refnum<class "RP Communicator.lvclass">)  [unwired: 7 in]
            n103 = Unbundle By Name(w261) -> ("fast_adc_1_1"=w260:T2, "fast_adc_1_20"=w259:T2)
            n104 = property class="RP Communicator.lvclass"(reference=w249, error in=w252) -> (reference out=w248:refnum<class "RP Communicator.lvclass">, error out=w250:errorcluster, "Accessors:Number of input channels"=w247:i32)
            n105 = Cluster To Array(cluster=w260) -> (array=w258:T3[])
            n106 = Cluster To Array(cluster=w259) -> (array=w257:T3[])
            n107 = local read "Input ranges"() -> (w254:bool[])
            n108 = for {
              N: w247 -> [_]
              tunnel: w258 -> [w269] mode=indexing
              tunnel: w257 -> [w268] mode=indexing
              tunnel: w254 -> [w267] mode=indexing
              tunnel: [w265] -> w251 mode=indexing
              tunnel: [w264] -> w253 mode=indexing
              n109 = Select(t=w269, s=w267, f=w268) -> (s? t:f=w266:T3)
              n110 = Unbundle By Name(w266) -> ("offset"=w264:i32, "gainCalc"=w265:dbl)
            }
            n111 = local write "In offsets"(w253) -> ()
            n112 = local write "In gains"(w251) -> ()
          }
        }
      }
      event "Stop calibration": Value Change {
        n113 = event-data() -> ()  [unwired: 1 in, 6 out]
        n114 = local write "Calibrating"(FALSE ("Calibrating")) -> ()
        n115 = call-dynamic "Close.vi"("error in (no error)"=w270, "RP Communicator in"=w272) -> ("error out"=w271:errorcluster, "RP Communicator out"=w273:refnum<class "RP Communicator.lvclass">)  [unwired: 8 in]
      }
      event "Find Red Pitayas": Value Change {
        n116 = event-data() -> ()  [unwired: 1 in, 6 out]
        n117 = call <vilib>:"Set Busy.vi"("error in (no error)"=w281) -> ("error out"=w280:errorcluster)  [unwired: 9 in, 1 out]
        n118 = call "Find Red Pitayas.vi"("Timeout"="Timeout", "Logic tags"=w289, "Error In"=w280, "End address"="End address", "Start address"="Start address", "Subnet"="Subnet") -> ("Error Out"=w285:errorcluster, "Addresses"=w284:string[], "Device names"=→"Device names":string[], "Modules"=→"Modules":i32[], "DDS modula out"=→"DDS modula out":i64[], "Logic tags out"=w288:u16[])
        "Logic tags out" <- w288
        "Addresses" <- w284
        n119 = for {
          tunnel: w288 -> [w325] mode=indexing
          tunnel: w287 -> [w326]
          tunnel: [w324] -> w286 mode=indexing
          shift-right: [w319] -> w278
          shift-left: w285 -> [w321]
          tunnel: w284 -> [w318] mode=indexing
          tunnel: [w316] -> w283 mode=indexing
          tunnel: [w311] -> w282 mode=indexing
          tunnel: "Board MAC address from eeprom: " -> [w304]
          tunnel: [w300] -> w275 mode=indexing
          w306 = "\r"
          w307 = "y" ("standard input")
          w301 = "\\n"
          n120 = Look In Map(map=w326, key=w325) -> (value=w324:string)  [unwired: 1 in, 1 out]
          n121 = Format Into String(format string="plink -pw changeme -no-antispoof root@%s \"/opt/bin/maglab_rp_info\"", error in=w321, w318) -> (resulting string=w308:string, error out=w320:errorcluster)  [unwired: 1 in]
          "command" <- w308
          n122 = Concatenate Strings(w307, w306, w307, w306) -> (w309:string)
          n123 = call <vilib>:"System Exec.vi"("run minimized? (F)"="minimized shell", "error in (no error)"=w320, "standard input"=w309, "command line"=w308) -> ("error out"=w319:errorcluster, "standard output"=w303:string)  [unwired: 4 in, 2 out]
          n124 = Match Pattern(string=w303, regular expression="Board name:\\s") -> (after substring=w305:string)  [unwired: 1 in, 3 out]
          n125 = Match Pattern(string=w303, regular expression="(rp_HPeZynqModels_t)") -> (after substring=w314:string)  [unwired: 1 in, 3 out]
          n126 = Match Pattern(string=w303, regular expression=w304) -> (after substring=w302:string)  [unwired: 1 in, 3 out]
          n127 = Match Pattern(string=w305, regular expression=w301) -> (before substring=w316:string)  [unwired: 1 in, 3 out]
          n128 = Match Pattern(string=w314, regular expression=w301) -> (before substring=w310:string)  [unwired: 1 in, 3 out]
          n129 = Decimal String To Number(string=w310) -> (number=w313:i32)  [unwired: 2 in, 1 out]
          n130 = Match Pattern(string=w302, regular expression=w301) -> (before substring=w300:string)  [unwired: 1 in, 3 out]
          n131 = Index Array(array=string[] ["7010", "7020"], index=w313) -> (element=w311:string)
        }
        n132 = Number To Decimal String(number=w288) -> (decimal integer string=w292:string[])  [unwired: 1 in]
        n133 = Build Array(w284, w283, w282, w292, w286, w275) -> (w291:string[][])
        n134 = call <vilib>:"Unset Busy.vi"("error in (no error)"=w278) -> ("error out"=w279:errorcluster)  [unwired: 10 in]
        n135 = Transpose 2D Array(2D array=w291) -> (transposed array=w290:string[][])
        n136 = property on="Red Pitayas" class="MCListbox (strict)"("ItemNames"=w290) -> ()  [unwired: 2 in, 2 out]
      }
      event "Calibration string": Value Change {
        n137 = event-data() -> ()  [unwired: 1 in, 6 out]
        n138 = Get Date/Time In Seconds() -> (seconds since 1Jan1904=w331:timestamp)
        n139 = local read "Out offsets"() -> (w340:i16[])
        n140 = local read "Out gains"() -> (w339:dbl[])
        n141 = local read "In gains"() -> (w341:dbl[])
        n142 = local read "In offsets"() -> (w342:i32[])
        n143 = Get Date/Time String(date format (0)=enum16{"short", "long", "abbreviated"}."short", seconds (now)=w331) -> (date string=w329:string)  [unwired: 1 in, 1 out]
        n144 = Concatenate Strings(w329, ": " ("string")) -> (w328:string)
        n145 = for {
          tunnel: w342 -> [w356] mode=indexing
          tunnel: w341 -> [w355] mode=indexing
          shift-right: [w352] -> w338
          shift-left: w328 -> [w353]
          shift-right: [w350] -> w334
          shift-left: w335 -> [w351]
          n146 = Format Into String(format string="%d, %f;", initial string=w353, error in=w351, w356, w355) -> (resulting string=w352:string, error out=w350:errorcluster)
        }
        n147 = for {
          tunnel: w340 -> [w349] mode=indexing
          tunnel: w339 -> [w348] mode=indexing
          shift-right: [w345] -> w337
          shift-left: w338 -> [w346]
          shift-right: [w343] -> w333
          shift-left: w334 -> [w344]
          n148 = Format Into String(format string="%d, %f;", initial string=w346, error in=w344, w349, w348) -> (resulting string=w345:string, error out=w343:errorcluster)
        }
        "String" <- w337
        n149 = invoke class="App" method="Clipboard.Write"(error in=w333, "Param 0"=w337) -> (error out=w332:errorcluster)  [unwired: 2 in, 3 out]
      }
      event Timeout {
        n150 = event-data() -> ()  [unwired: 1 in, 3 out]
        n151 = local read "Calibrating"() -> (w361:bool)
        n152 = case shown="False" w361 {
          tunnel: w360 -> [w363 w382]
          tunnel: [w363 w376] -> w359
          tunnel: w358 -> [w362 w386]
          tunnel: [w362 w377] -> w357
          frame False {
          }
          frame True {
            n153 = property class="RP Communicator.lvclass"(reference=w386, error in=w382) -> (reference out=w384:refnum<class "RP Communicator.lvclass">, error out=w383:errorcluster, "Accessors:Number of input channels"=w385:i32, "Accessors:Logic tag"=w372:u16, "Accessors:Input ranges"=w365:bool[])
            n154 = call "RP Logic Specs.vi"("Logic tag"=w372) -> ("DC Gain"=w370:dbl, "DC address increment"=w367:i32)  [unwired: 4 in, 5 out]
            n155 = for {
              N: w385 -> [_]
              shift-right: [w401] -> w377
              shift-left: w384 -> [w402]
              shift-right: [w394] -> w376
              shift-left: w383 -> [w395]
              tunnel: [w392] -> w381 mode=indexing
              tunnel: w367 -> [w391]
              tunnel: w365 -> [w388] mode=indexing
              tunnel: [w387] -> w364 mode=indexing
              i -> [w400]
              n156 = Multiply(x=w400, y=w391) -> (x*y=w398:i32)
              n157 = Add(x=16, y=w398) -> (x+y=w397:i32)
              n158 = To Unsigned Quad Integer(1:w397) -> (0:w396:u64)
              n159 = call-dynamic "Recieve Status.vi"("error in (no error)"=w395, "Status offset"=w396, "RP Communicator in"=w402) -> ("error out"=w394:errorcluster, "Status response"=w393:u32, "RP Communicator out"=w401:refnum<class "RP Communicator.lvclass">)  [unwired: 6 in]
              n160 = To Long Integer(number=w393) -> (32bit integer=w392:i32)
              n161 = Select(t=20.0, s=w388, f=1.0 ("t")) -> (s? t:f=w387:dbl)
            }
            n162 = Multiply(x=w370, y=8192.0) -> (x*y=w368:dbl)
            n163 = Divide(x="In offsets", y=w368) -> (x/y=w374:dbl[])
            n164 = Subtract(x=w381, y=w374) -> (x-y=w371:dbl[])
            n165 = Multiply(x=w370, y=w371) -> (x*y=w380:dbl[])
            n166 = Multiply(x="In gains", y=w380) -> (x*y=w378:dbl[])
            n167 = Multiply(x=w378, y=w364) -> (x*y=w366:dbl[])
            n168 = Build Array(w366) -> (→"Waveform Chart":dbl[][])
          }
        }
      }
      event "Auto offsets": Value Change {
        n169 = event-data() -> ()  [unwired: 1 in, 6 out]
        n170 = local read "Calibrating"() -> (w405:bool)
        n171 = case shown="True" w405 {
          tunnel: w403 -> [_ w415]
          frame False {
          }
          frame True {
            n172 = local read "Waveform Chart"() -> (w416:dbl[][])
            n173 = property class="RP Communicator.lvclass"(reference=w415) -> ("Accessors:Input ranges"=w406:bool[], "Accessors:Number of input channels"=w414:i32)  [unwired: 1 in, 2 out]
            n174 = Index Array(array=w416, index (row)=0) -> (element=w413:dbl[])  [unwired: 1 in]
            n175 = local read "In gains"() -> (w412:dbl[])
            n176 = for {
              N: w414 -> [_]
              tunnel: w413 -> [w427] mode=indexing
              tunnel: w412 -> [w426] mode=indexing
              tunnel: 8192.0 ("y") -> [w425]
              tunnel: [w420] -> w409 mode=indexing
              tunnel: w406 -> [w423] mode=indexing
              n177 = Select(t=20.0, s=w423, f=1.0 ("t")) -> (s? t:f=w418:dbl)
              n178 = Multiply(x=w418, y=w426) -> (x*y=w419:dbl)
              n179 = Divide(x=w427, y=w419) -> (x/y=w424:dbl)
              n180 = Multiply(x=w424, y=w425) -> (x*y=w420:dbl)
            }
            n181 = local read "In offsets"() -> (w410:i32[])
            n182 = To Long Integer(number=w409) -> (32bit integer=w408:i32[])
            n183 = Add(x=w410, y=w408) -> (x+y=w407:i32[])
            n184 = local write "In offsets"(w407) -> ()
          }
        }
      }
      event "Auto gains": Value Change {
        n185 = event-data() -> ()  [unwired: 1 in, 6 out]
        n186 = local read "Calibrating"() -> (w429:bool)
        n187 = case shown="True" w429 {
          tunnel: w428 -> [_ w437]
          frame False {
          }
          frame True {
            n188 = property class="RP Communicator.lvclass"(reference=w437) -> ("Accessors:Input ranges"=w432:bool[])  [unwired: 1 in, 2 out]
            n189 = local read "Waveform Chart"() -> (w439:dbl[][])
            n190 = for {
              tunnel: w432 -> [w441] mode=indexing
              tunnel: [w440] -> _ mode=indexing
              n191 = Select(t=20.0, s=w441, f=1.0 ("t")) -> (s? t:f=w440:dbl)
            }
            n192 = local read "In gains"() -> (w433:dbl[])
            n193 = Index Array(array=w439, index (row)=0) -> (element=w435:dbl[])  [unwired: 1 in]
            n194 = Divide(x=w435, y=w433) -> (x/y=w434:dbl[])
            n195 = Divide(x="Applied \nvoltage", y=w434) -> (x/y=w431:dbl[])
            n196 = local write "In gains"(w431) -> ()
          }
        }
      }
      event "View  bitfiles": Value Change {
        n197 = event-data() -> ()  [unwired: 1 in, 6 out]
        n198 = property on="Red Pitayas" class="MCListbox (strict)"() -> ("ItemNames"=w457:string[][])  [unwired: 2 in, 2 out]
        n199 = Index Array(array=w457, index (row)="Red Pitayas", index (col)=0 ("disabled index (col)")) -> (element=w453:string)
        n200 = call <vilib>:"Set Busy.vi"("error in (no error)"=w454) -> ("error out"=w445:errorcluster)  [unwired: 9 in, 1 out]
        n201 = Format Into String(format string="plink -pw changeme -no-antispoof root@%s \"ls /opt\" ", error in=w445, w453) -> (resulting string=w460:string, error out=w458:errorcluster)  [unwired: 1 in]
        n202 = call <vilib>:"System Exec.vi"("run minimized? (F)"=TRUE, "error in (no error)"=w458, "command line"=w460) -> ("error out"=w446:errorcluster, "standard output"=w449:string)  [unwired: 5 in, 2 out]
        n203 = while {
          shift-right: [w465] -> w450
          shift-left: "" -> [w471]
          shift-right: [w469] -> w447
          shift-left: w446 -> [w468]
          shift-right: [w467] -> _
          shift-left: 0 ("offset past match") -> [w466]
          tunnel: w449 -> [w462]
          stop <- w463 stop-if-true
          n204 = xnode "Match Regular Expression"("input string"=w462, "regular expression"="(?m)^\\S.*?\\.bit", "offset (0)"=w466, "error in"=w468) -> ("whole match"=w464:string, "offset past match"=w467:i32, "error out"=w469:errorcluster)  [unwired: 2 in, 2 out]
          n205 = Empty String/Path?(string/path=w464) -> (empty?=w463:bool)
          n206 = Concatenate Strings(w471, w464, "\r\n") -> (w465:string)
        }
        "bit files" <- w450
        n207 = call <vilib>:"Unset Busy.vi"("error in (no error)"=w447) -> ("error out"=w444:errorcluster)  [unwired: 10 in]
      }
      event "View  startup": Value Change {
        n208 = event-data() -> ()  [unwired: 1 in, 6 out]
        n209 = call <vilib>:"Set Busy.vi"("error in (no error)"=w596) -> ("error out"=w591:errorcluster)  [unwired: 9 in, 1 out]
        n210 = property on="Red Pitayas" class="MCListbox (strict)"() -> ("ItemNames"=w597:string[][], "Value"=w595:i32)  [unwired: 2 in, 2 out]
        n211 = Index Array(array=w597, index (row)=w595, index (col)=0 ("disabled index (col)")) -> (element=w598:string)
        n212 = Format Into String(format string="plink -pw changeme -no-antispoof root@%s \"cat /opt/bin/start_rp.sh \" ", error in=w591, w598) -> (resulting string=w602:string, error out=w600:errorcluster)  [unwired: 1 in]
        n213 = call <vilib>:"System Exec.vi"("run minimized? (F)"=TRUE, "error in (no error)"=w600, "command line"=w602) -> ("error out"=w593:errorcluster, "standard output"=→"Starup script":string)  [unwired: 5 in, 2 out]
        n214 = call <vilib>:"Unset Busy.vi"("error in (no error)"=w593) -> ("error out"=w590:errorcluster)  [unwired: 10 in]
      }
    }
    n215 = Or(x=w27, y=w26) -> (x .or. y?=w25:bool)
  }
  n216 = call <vilib>:"Simple Error Handler.vi"("error in (no error)"=w6) -> ()  [unwired: 4 in, 5 out]
